vi "Compute_trap_PID.vi"(0 "Final Position [Rad]":dbl=1000.0, 1 "Vcruise [Rad/s]":dbl=200.0, 2 "Kp":T1={"proportional gain (Kc)"=1.5, "integral time (Ti, min)"=0.0, "derivative time (Td, min)"=0.0} {"derivative time (Td, min)" format="%.3f"; "integral time (Ti, min)" format="%.3f"; "proportional gain (Kc)" format="%.3f"}, 3 "Kv":T1={"proportional gain (Kc)"=0.0006, "integral time (Ti, min)"=0.0005, "derivative time (Td, min)"=0.0} {"derivative time (Td, min)" format="%.3f"; "integral time (Ti, min)" format="%.3e"; "proportional gain (Kc)" format="%.3e"}, 5 "Acceleration [Rad/s^2]":dbl=100.0, 7 "Deceleration [Rad/s^2]":dbl=100.0, 9 "MinFrac_Cruise":dbl=0.3, 11 "Current Time":dbl, 12 "P_fb":dbl format="%.2f", 14 "V_fb":dbl format="%.2f") -> (4 "vSetProfile":dbl, 6 "PWM Signal":dbl format="%.2f", 8 "pSetProfile":dbl, 15 "vFeedforward":dbl format="%.2f")   [LabVIEW 2014]
uses:
  <vilib>/addons/control/pid/pid.llb/PID (DBL).vi
  <vilib>/addons/control/pid/NI_PID_pid.lvlib
panel:
  out "V_cruise":dbl
  in  "Init_Position [Rad]":dbl
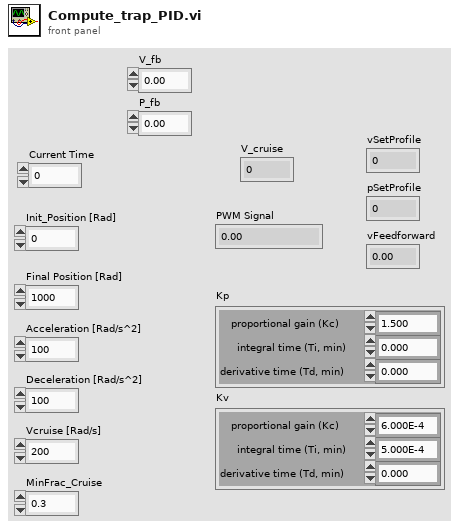
[diagram p1: front panel]
types:
  T1 = cluster{"proportional gain (Kc)":dbl, "integral time (Ti, min)":dbl, "derivative time (Td, min)":dbl}
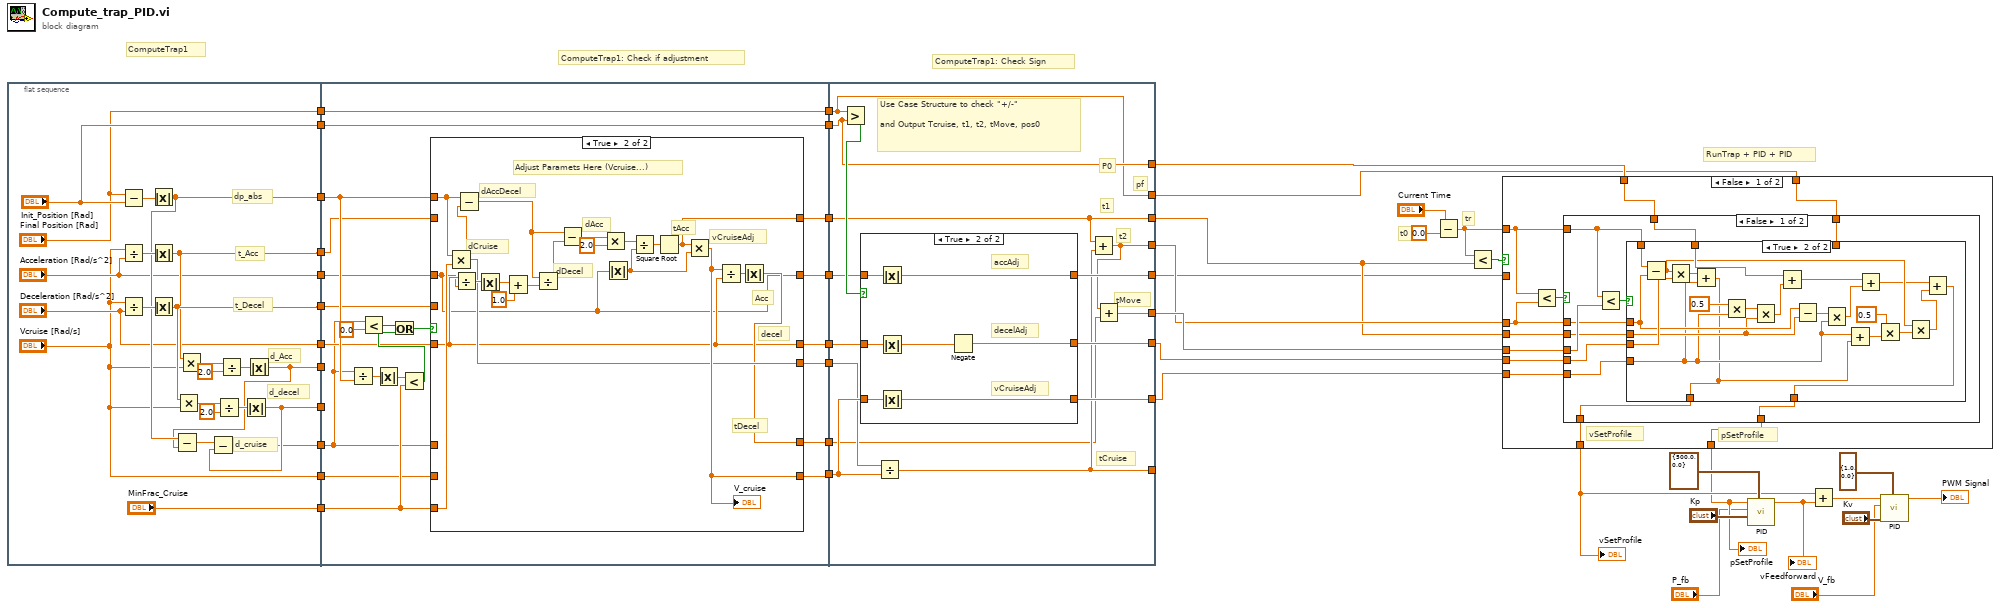
[diagram p0: block diagram]
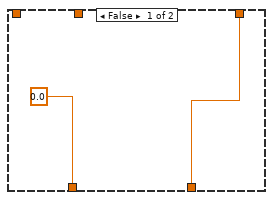
[diagram p2: hidden frame]
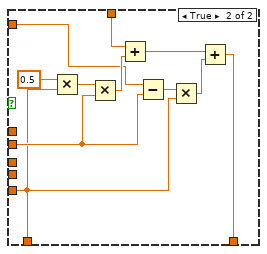
[diagram p3: hidden frame]
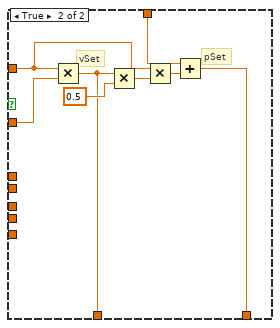
[diagram p4: hidden frame]
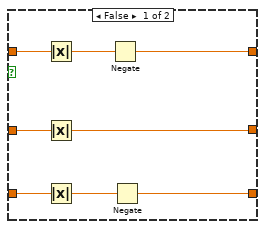
[diagram p6: hidden frame]
diagram:
  # "tr"
  # "t0"
  # "RunTrap + PID + PID"
  # "ComputeTrap1: Check Sign"
  # "ComputeTrap1: Check if adjustment"
  # "ComputeTrap1"
  n1 = flat-sequence {
    tunnel: [w55] -> w43
    tunnel: [w51] -> w42
    tunnel: [w54] -> w41
    tunnel: [w53] -> w40
    tunnel: [w52] -> w39
    tunnel: [w44] -> w38
    tunnel: ["MinFrac_Cruise"] -> w37
    tunnel: ["Acceleration [Rad/s^2]"] -> w36
    tunnel: ["Deceleration [Rad/s^2]"] -> w35
    tunnel: ["Vcruise [Rad/s]"] -> w34
    tunnel: ["Init_Position [Rad]"] -> w33
    tunnel: ["Final Position [Rad]"] -> w32
    tunnel: w43 -> [w80]
    tunnel: w42 -> [w76]
    tunnel: w41 -> [w66]
    tunnel: w40 -> [_]
    tunnel: w39 -> [_]
    tunnel: w38 -> [w75]
    tunnel: w37 -> [w81]
    tunnel: w36 -> [w79]
    tunnel: w35 -> [w78]
    tunnel: w34 -> [w77]
    tunnel: [w74] -> w31
    tunnel: [w73] -> w30
    tunnel: [w72] -> w29
    tunnel: [w71] -> w28
    tunnel: [w70] -> w27
    tunnel: w33 -> [w69]
    tunnel: [w69] -> w26
    tunnel: w32 -> [w68]
    tunnel: [w68] -> w25
    tunnel: [w67] -> w24
    tunnel: w31 -> [w119]
    tunnel: w30 -> [w127]
    tunnel: w29 -> [w126]
    tunnel: w28 -> [w120]
    tunnel: w27 -> [w121]
    tunnel: w26 -> [w122]
    tunnel: w25 -> [w114]
    tunnel: [w125] -> w16
    tunnel: [w124] -> w22
    tunnel: [w123] -> w23
    tunnel: [w122] -> w19
    tunnel: [w118] -> _
    tunnel: [w119] -> w17
    tunnel: [w116] -> w20
    tunnel: w24 -> [w117]
    tunnel: [w115] -> w21
    tunnel: [w114] -> w18
    frame #0 {
      # "d_cruise"
      # "d_decel"
      # "d_Acc"
      # "t_Decel"
      # "t_Acc"
      # "dp_abs"
      n2 = Subtract(x="Final Position [Rad]", y="Init_Position [Rad]") -> (x-y=w56:dbl)
      n3 = Divide(x="Vcruise [Rad/s]", y="Acceleration [Rad/s^2]") -> (x/y=w57:dbl)
      n4 = Divide(x="Vcruise [Rad/s]", y="Deceleration [Rad/s^2]") -> (x/y=w58:dbl)
      n5 = Absolute Value(x=w56) -> (abs(x)=w55:dbl)
      n6 = Absolute Value(x=w57) -> (abs(x)=w51:dbl)
      n7 = Absolute Value(x=w58) -> (abs(x)=w54:dbl)
      n8 = Multiply(x=w54, y="Vcruise [Rad/s]") -> (x*y=w64:dbl)
      n9 = Multiply(x=w51, y="Vcruise [Rad/s]") -> (x*y=w59:dbl)
      n10 = Divide(x=w64, y=2.0) -> (x/y=w62:dbl)
      n11 = Divide(x=w59, y=2.0) -> (x/y=w61:dbl)
      n12 = Absolute Value(x=w62) -> (abs(x)=w52:dbl)
      n13 = Absolute Value(x=w61) -> (abs(x)=w53:dbl)
      n14 = Subtract(x=w55, y=w53) -> (x-y=w65:dbl)
      n15 = Subtract(x=w65, y=w52) -> (x-y=w44:dbl)
    }
    frame #1 {
      n16 = Divide(x=w75, y=w80) -> (x/y=w84:dbl)
      n17 = Less?(x=w75, y=0.0) -> (x < y?=w85:bool)
      n18 = Absolute Value(x=w84) -> (abs(x)=w83:dbl)
      n19 = Less?(x=w83, y=w81) -> (x < y?=w82:bool)
      n20 = Or(x=w85, y=w82) -> (x .or. y?=w86:bool)
      n21 = case shown="True" w86 {
        tunnel: w81 -> [_ w113]
        tunnel: w80 -> [_ w112]
        tunnel: w79 -> [w90 w94]
        tunnel: w78 -> [w89 w95]
        tunnel: w77 -> [w93 _]
        tunnel: [w93 w99] -> w70
        tunnel: [w92 w98] -> w74
        tunnel: [w91 w97] -> w71
        tunnel: w76 -> [w92 _]
        tunnel: w75 -> [w91 _]
        tunnel: [w90 w94] -> w73
        tunnel: [w89 w95] -> w72
        tunnel: [w88 w96] -> w67
        tunnel: w66 -> [w88 _]
        frame False {
          # "t_Decel"
          # "Decel"
          # "Acc"
          # "d_Cruise"
          # "t_Acc"
          # "vCruiseAdj"
          # "vCruiseAdj = vCruise"
        }
        frame True {
          # "Acc"
          # "decel"
          # "tDecel"
          # "vCruiseAdj"
          # "tAcc"
          # "dAcc"
          # "dDecel"
          # "dAccDecel"
          # "dCruise"
          # "Adjust Paramets Here (Vcruise...)"
          n22 = Multiply(x=w112, y=w113) -> (x*y=w97:dbl)
          n23 = Divide(x=w95, y=w94) -> (x/y=w111:dbl)
          n24 = Subtract(x=w112, y=w97) -> (x-y=w106:dbl)
          n25 = Absolute Value(x=w111) -> (abs(x)=w110:dbl)
          n26 = Add(x=w110, y=1.0) -> (x+y=w108:dbl)
          n27 = Divide(x=w106, y=w108) -> (x/y=w107:dbl)
          n28 = Subtract(x=w106, y=w107) -> (x-y=w105:dbl)
          n29 = Multiply(x=w105, y=2.0) -> (x*y=w103:dbl)
          n30 = Absolute Value(x=w94) -> (abs(x)=w101:dbl)
          n31 = Divide(x=w103, y=w101) -> (x/y=w102:dbl)
          n32 = Square Root(x=w102) -> (sqrt(x)=w98:dbl)
          n33 = Multiply(x=w98, y=w101) -> (x*y=w99:dbl)
          "V_cruise" <- w99
          n34 = Divide(x=w99, y=w95) -> (x/y=w100:dbl)
          n35 = Absolute Value(x=w100) -> (abs(x)=w96:dbl)
        }
      }
    }
    frame #2 {
      # "pf"
      # "tMove"
      # "t2"
      # "t1"
      # "tCruise"
      # "P0"
      # "Use Case Structure to check \"+/-\"\n\nand Output Tcruise, t1, t2, tMove, pos0"
      n36 = Greater?(x=w114, y=w122) -> (0:w128:bool)
      n37 = case shown="True" w128 {
        tunnel: w127 -> [w136 w143]
        tunnel: w126 -> [w135 w142]
        tunnel: w121 -> [w134 w141]
        tunnel: [w132 w140] -> w125
        tunnel: [w129 w139] -> w123
        tunnel: [w131 w137] -> w124
        frame False {
          n38 = Absolute Value(x=w136) -> (abs(x)=w133:dbl)
          n39 = Absolute Value(x=w135) -> (abs(x)=w131:dbl)
          n40 = Absolute Value(x=w134) -> (abs(x)=w130:dbl)
          n41 = Negate(x=w133) -> (-x=w132:dbl)
          n42 = Negate(x=w130) -> (-x=w129:dbl)
        }
        frame True {
          # "vCruiseAdj"
          # "decelAdj"
          # "accAdj"
          n43 = Absolute Value(x=w143) -> (abs(x)=w140:dbl)
          n44 = Absolute Value(x=w142) -> (abs(x)=w138:dbl)
          n45 = Absolute Value(x=w141) -> (abs(x)=w139:dbl)
          n46 = Negate(x=w138) -> (-x=w137:dbl)
        }
      }
      n47 = Divide(x=w120, y=w121) -> (x/y=w118:dbl)
      n48 = Add(x=w119, y=w118) -> (x+y=w116:dbl)
      n49 = Add(x=w116, y=w117) -> (x+y=w115:dbl)
    }
  }
  n50 = Subtract(x="Current Time", y=0.0) -> (x-y=w13:dbl)
  n51 = Less?(x=w13, y=w17) -> (x < y?=w14:bool)
  n52 = case shown="False" w14 {
    tunnel: w16 -> [_ w207]
    tunnel: w13 -> [w149 w204]
    tunnel: w19 -> [w151 w202]
    tunnel: [w148 w201] -> w4
    tunnel: [w152 w200] -> w6
    tunnel: w20 -> [w144 _]
    tunnel: w23 -> [w153 _]
    tunnel: w17 -> [w150 _]
    tunnel: w21 -> [w147 _]
    tunnel: w18 -> [w146 _]
    tunnel: w22 -> [w145 _]
    frame False {
      # "pSetProfile"
      # "vSetProfile"
      n53 = Less? ("Less? 2")(x=w149, y=w144) -> (x < y?=w154:bool)
      n54 = case "Case Structure 2" shown="False" w154 {
        tunnel: w153 -> [w160 w191]
        tunnel: [w163 w191] -> w152
        tunnel: w151 -> [w156 w199]
        tunnel: w150 -> [w155 w193]
        tunnel: w149 -> [w159 w194]
        tunnel: [w161 w189] -> w148
        tunnel: w147 -> [w164 _]
        tunnel: w146 -> [w162 _]
        tunnel: w145 -> [w157 _]
        tunnel: w144 -> [w158 _]
        frame False {
          n55 = Less? ("Less? 3")(x=w159, y=w164) -> (x < y?=w165:bool)
          n56 = case "Case Structure 3" shown="True" w165 {
            tunnel: [0.0 ("y 3") w175] -> w163
            tunnel: [w166 w168] -> w161
            tunnel: w162 -> [w166 _]
            tunnel: w160 -> [_ w176]
            tunnel: w159 -> [_ w182]
            tunnel: w158 -> [_ w178]
            tunnel: w157 -> [_ w181]
            tunnel: w156 -> [_ w179]
            tunnel: w155 -> [_ w177]
            frame False {
            }
            frame True {
              n57 = Subtract ("Subtract 4")(x=w182, y=w178) -> (x-y=w171:dbl)
              n58 = Multiply ("Multiply 10")(x=w171, y=w181) -> (x*y=w180:dbl)
              n59 = Add ("Add 6")(x=w180, y=w176) -> (x+y=w175:dbl)
              n60 = Multiply ("Multiply 7")(x=0.5 ("x 2"), y=w176) -> (x*y=w187:dbl)
              n61 = Multiply ("Multiply 8")(x=w187, y=w177) -> (x*y=w186:dbl)
              n62 = Add ("Add 4")(x=w179, y=w186) -> (x+y=w185:dbl)
              n63 = Subtract ("Subtract 3")(x=w178, y=w177) -> (x-y=w184:dbl)
              n64 = Multiply ("Multiply 9")(x=w184, y=w176) -> (x*y=w183:dbl)
              n65 = Add ("Add 7")(x=w176, y=w175) -> (x+y=w174:dbl)
              n66 = Add ("Add 5")(x=w185, y=w183) -> (x+y=w170:dbl)
              n67 = Multiply ("Multiply 11")(x=0.5 ("x 3"), y=w174) -> (x*y=w172:dbl)
              n68 = Multiply ("Multiply 12")(x=w171, y=w172) -> (x*y=w169:dbl)
              n69 = Add ("Add 8")(x=w170, y=w169) -> (x+y=w168:dbl)
            }
          }
        }
        frame True {
          n70 = Multiply ("Multiply 4")(x=0.5, y=w191) -> (x*y=w197:dbl)
          n71 = Multiply ("Multiply 5")(x=w197, y=w193) -> (x*y=w196:dbl)
          n72 = Add ("Add 2")(x=w199, y=w196) -> (x+y=w195:dbl)
          n73 = Subtract ("Subtract 2")(x=w194, y=w193) -> (x-y=w192:dbl)
          n74 = Multiply ("Multiply 6")(x=w192, y=w191) -> (x*y=w190:dbl)
          n75 = Add ("Add 3")(x=w195, y=w190) -> (x+y=w189:dbl)
        }
      }
    }
    frame True {
      # "pSet"
      # "vSet"
      n76 = Multiply(x=w204, y=w207) -> (x*y=w200:dbl)
      n77 = Multiply ("Multiply 2")(x=w200, y=0.5 ("y 2")) -> (x*y=w205:dbl)
      n78 = Multiply ("Multiply 3")(x=w204, y=w205) -> (x*y=w203:dbl)
      n79 = Add(x=w202, y=w203) -> (x+y=w201:dbl)
    }
  }
  "vSetProfile" <- w6
  "pSetProfile" <- w4
  n80 = call-poly <vilib>:"PID.vi"("output range"=cluster{"output high":dbl, "output low":dbl} {"output high"=500.0, "output low"=0.0}, "PID gains"="Kp", "process variable"="P_fb", "setpoint"=w4) -> ("output"=w11:dbl)  [unwired: 6 in, 1 out]
  "vFeedforward" <- w11
  n81 = Add(x=w6, y=w11) -> (x+y=w5:dbl)
  n82 = call-poly <vilib>:"PID.vi"("output range"=cluster{"output high":dbl, "output low":dbl} {"output high"=1.0, "output low"=0.0}, "PID gains"="Kv", "process variable"="V_fb", "setpoint"=w5) -> ("output"=→"PWM Signal":dbl)  [unwired: 6 in, 1 out]
